vi "Move(X)feet.vi"(3 "Target":dbl, 5 "RobotDriveDevRef":T1={"DevStatus"={"status"=FALSE, "code"=0, "source"=""}, "Motors[]"=[], "Square Inputs"=FALSE, "Max Output"=1.0}, 6 "AccelerometerDevRef":T7={"DevStatus"={"status"=FALSE, "code"=0, "source"=""}, "Scaling"={"Gain (VoltsPerG)"=0.0, "Center Voltage"=0.0}, "Analog Channels"={"X-Axis"=enum."Invalid", "Y-Axis"=enum."Invalid", "Z-Axis"=enum."Invalid"}, "I2C Bus"=enum."Invalid", "SPI Bus"=enum."Invalid", "Accel Range"=0, "ADXL Axes"={"X-Axis"=FALSE, "Y-Axis"=FALSE, "Z-Axis"=FALSE}, "Handle"=0, "Device Address"=0, "Accel Type"=enum."Analog"} {"Device Address" format="%.0x"; "Accel Range" items=["+/- 2 g", "+/- 4 g", "+/- 8 g", "+/- 16 g"]}) -> (1 "RobotDriveDevRef":T1={"DevStatus"={"status"=FALSE, "code"=0, "source"=""}, "Motors[]"=[], "Square Inputs"=FALSE, "Max Output"=1.0}, 2 "AccelerometerDevRef":T7={"DevStatus"={"status"=FALSE, "code"=0, "source"=""}, "Scaling"={"Gain (VoltsPerG)"=0.0, "Center Voltage"=0.0}, "Analog Channels"={"X-Axis"=enum."Invalid", "Y-Axis"=enum."Invalid", "Z-Axis"=enum."Invalid"}, "I2C Bus"=enum."Invalid", "SPI Bus"=enum."Invalid", "Accel Range"=0, "ADXL Axes"={"X-Axis"=FALSE, "Y-Axis"=FALSE, "Z-Axis"=FALSE}, "Handle"=0, "Device Address"=0, "Accel Type"=enum."Analog"} {"Device Address" format="%.0x"; "Accel Range" items=["+/- 2 g", "+/- 4 g", "+/- 8 g", "+/- 16 g"]})   [LabVIEW 2017]
uses:
  <vilib>/Rock Robotics/WPI/Accelerometer/WPI_AccelerometerDevRef.ctl
  <vilib>/Rock Robotics/WPI/Accelerometer/WPI_AccelerometerScaling.ctl
  <vilib>/Rock Robotics/WPI/Accelerometer/WPI_AccelerometerAnalogChannels.ctl
  <vilib>/Rock Robotics/SystemInterfaces/AI/FPGA_AIChannel.ctl
  <vilib>/Rock Robotics/SystemInterfaces/i2clib/i2c_bus.ctl
  <vilib>/Rock Robotics/SystemInterfaces/spilib/spi_bus.ctl
  <vilib>/Rock Robotics/WPI/Accelerometer/ADXL345 Range.ctl
  <vilib>/Rock Robotics/WPI/Accelerometer/WPI_AccelerometerADXL345 Axes.ctl
  <vilib>/Rock Robotics/WPI/RobotDrive/WPI_RobotDriveDevRef.ctl
  <vilib>/Rock Robotics/WPI/MotorControl/WPI_MotorControlDeviceRef.ctl
  <vilib>/Rock Robotics/WPI/MotorControl/WPI_MotorControlType.ctl
  <vilib>/Rock Robotics/SystemInterfaces/DIO/FPGA_DIOPWMChannel.ctl
  <vilib>/Rock Robotics/WPI/PWM/WPI_PWMDeadband.ctl
  <vilib>/Rock Robotics/SystemInterfaces/DIO/FPGA_DIOChannel.ctl
  <vilib>/Rock Robotics/WPI/RobotDrive/WPI_RobotDriveArcadeDrive_Standard(NoSaturation).vi
  <vilib>/Rock Robotics/Network Tables/NT Write Number.vi
  <vilib>/Rock Robotics/Network Tables/NT Write Numeric Array.vi
panel:
  in  "Speed":dbl
  in  "Velocity":dbl
  in  "Distance":dbl
  in  "Start Time":dbl
  # "ADXL"
  # "Analog"
  # "ADXL"
  # "Analog"
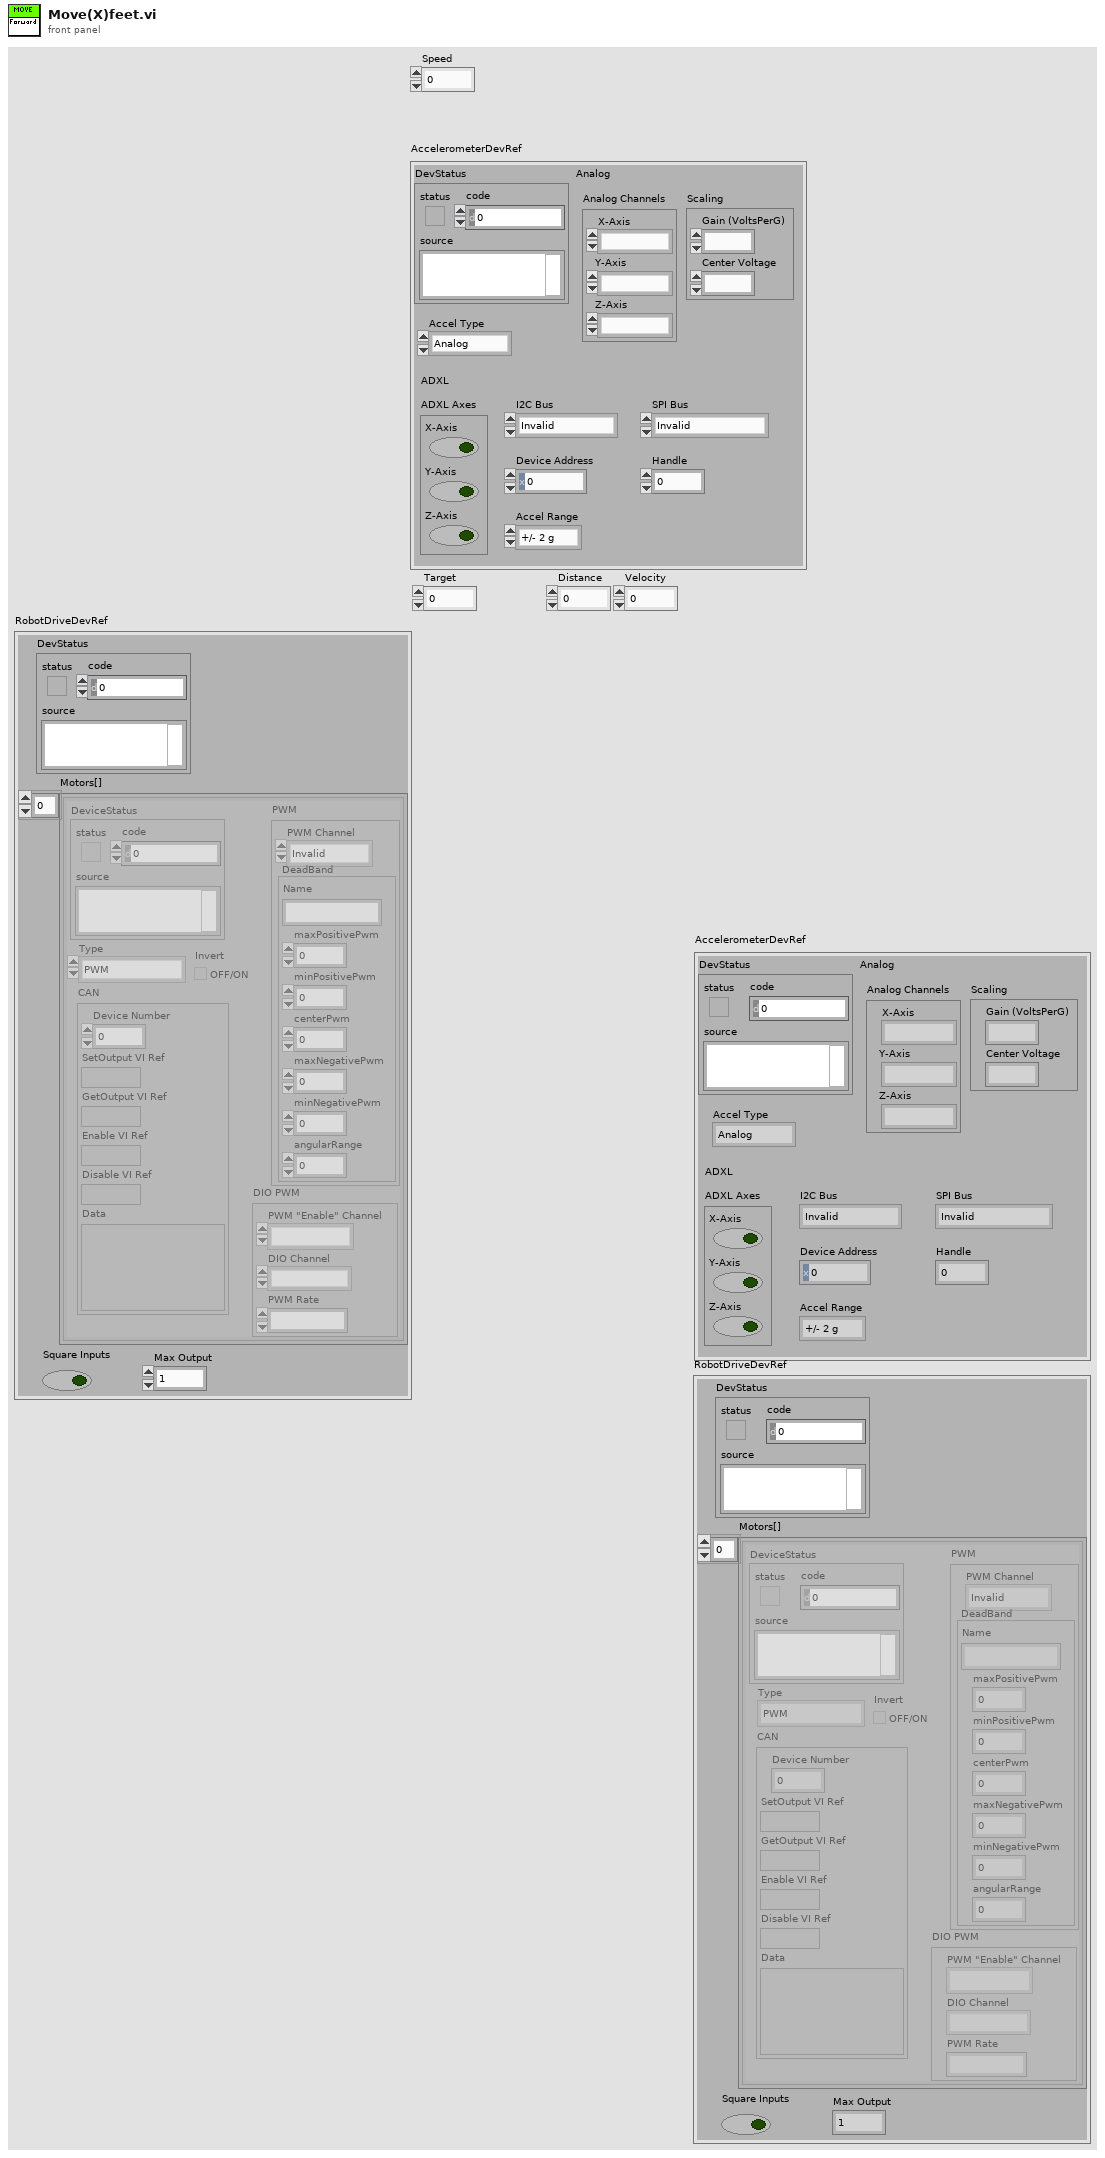
[diagram p1: front panel]
types:
  T1 = typedef "WPI_RobotDriveDevRef.ctl" = cluster{"DevStatus":errorcluster, "Motors[]":T2[], "Square Inputs":bool, "Max Output":dbl}
  T2 = typedef "WPI_MotorControlDeviceRef.ctl" = cluster{"DeviceStatus":errorcluster, "Type":T3, "PWM":cluster{"PWM Channel":T4, "DeadBand":T5}, "CAN":cluster{"Device Number":u8, "SetOutput VI Ref":variant, "GetOutput VI Ref":variant, "Enable VI Ref":variant, "Disable VI Ref":variant, "Data":variant}, "Invert":bool, "DIO PWM":cluster{"PWM \"Enable\" Channel":T4, "DIOChannel":T6, "PWM Rate":dbl}}
  T3 = typedef "WPI_MotorControlType.ctl" = enum16{"PWM", "CAN", "DIO PWM"}
  T4 = typedef "FPGA_DIOPWMChannel.ctl" = enum8{"PWM 0", "PWM 1", "PWM 2", "PWM 3", "PWM 4", "PWM 5", "PWM 6", "PWM 7", "PWM 8", "PWM 9", "PWM MXP 0", "PWM MXP 1", "PWM MXP 2", "PWM MXP 3", "PWM MXP 4", "PWM MXP 5", "PWM MXP 6", "PWM MXP 7", "PWM MXP 8", "PWM MXP 9", "Invalid"}
  T5 = typedef "WPI_PWMDeadband.ctl" = cluster{"Name":string, "maxPositivePwm":i32, "minPositivePwm":i32, "centerPwm":i32, "maxNegativePwm":i32, "minNegativePwm":i32, "angularRange":u16}
  T6 = typedef "FPGA_DIOChannel.ctl" = enum8{"DIO 0", "DIO 1", "DIO 2", "DIO 3", "DIO 4", "DIO 5", "DIO 6", "DIO 7", "DIO 8", "DIO 9", "DIO MXP 0", "DIO MXP 1", "DIO MXP 2", "DIO MXP 3", "DIO MXP 4", "DIO MXP 5", "DIO MXP 6", "DIO MXP 7", "DIO MXP 8", "DIO MXP 9", "DIO MXP 10", "DIO MXP 11", "DIO MXP 12", "DIO MXP 13", "DIO MXP 14", "DIO MXP 15", "SPI Port CS1", "SPI Port CS2", "SPI Port CS3", "SPI Port MISO", "SPI Port MOSI", "Invalid"}
  T7 = typedef "WPI_AccelerometerDevRef.ctl" = cluster{"DevStatus":errorcluster, "Scaling":T8, "Analog Channels":T9, "I2C Bus":T11, "SPI Bus":T12, "Accel Range":T13, "ADXL Axes":T14, "Handle":i32, "Device Address":u8, "Accel Type":enum16{"Analog", "ADXL345 I2C", "ADXL345 SPI", "Internal", "ADXL362 SPI"}}
  T8 = typedef "WPI_AccelerometerScaling.ctl" = cluster{"Gain (VoltsPerG)":dbl, "Center Voltage":dbl}
  T9 = typedef "WPI_AccelerometerAnalogChannels.ctl" = cluster{"X-Axis":T10, "Y-Axis":T10, "Z-Axis":T10}
  T10 = typedef "FPGA_AIChannel.ctl" = enum8{"AI 0", "AI 1", "AI 2", "AI 3", "AI MXP 0", "AI MXP 1", "AI MXP 2", "AI MXP 3", "Invalid"}
  T11 = typedef "i2c_bus.ctl" = enum16{"I2C On-Board", "I2C MXP", "Invalid"}
  T12 = typedef "spi_bus.ctl" = enum16{"SPI On-Board, CS0", "SPI On-Board, CS1", "SPI On-Board, CS2", "SPI On-Board, CS3", "SPI MXP", "Invalid"}
  T13 = typedef "ADXL345 Range.ctl" = u8
  T14 = typedef "WPI_AccelerometerADXL345 Axes.ctl" = cluster{"X-Axis":bool, "Y-Axis":bool, "Z-Axis":bool}
  T15 = cluster{"X-Axis":dbl, "Y-Axis":dbl, "Z-Axis":dbl}
  T16 = cluster{"Target":dbl, "Distance":dbl, dbl, dbl, dbl}
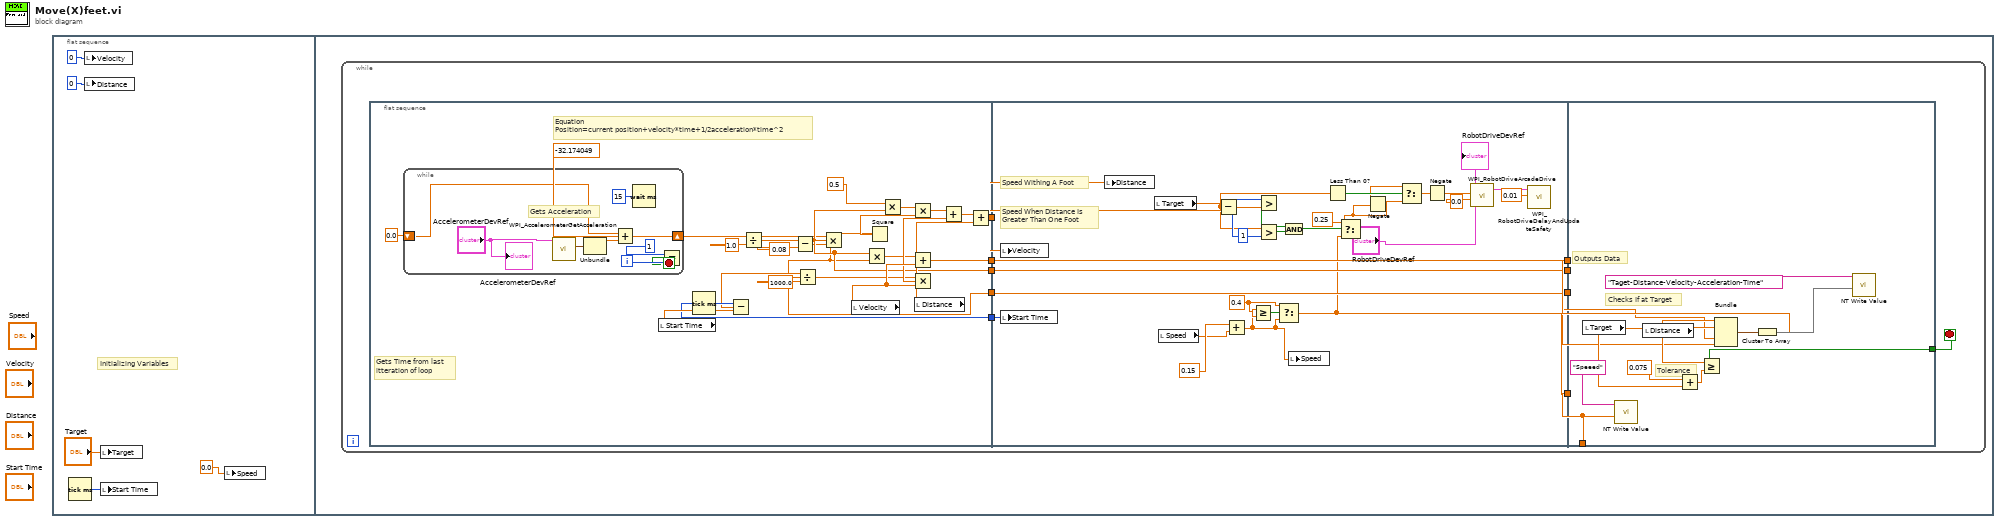
[diagram p0: block diagram]
diagram:
  n1 = flat-sequence {
    frame #0 {
      # "Initializing Variables"
      n2 = Tick Count (ms)() -> (millisecond timer value=w5:u32)
      n3 = local write "Velocity"(0) -> ()
      n4 = local write "Distance"(0) -> ()
      n5 = local write "Target"("Target") -> ()
      n6 = local write "Start Time"(w5) -> ()
      n7 = local write "Speed"(0.0) -> ()
    }
    frame #1 {
      n8 = while {
        stop <- w12 stop-if-true
        n9 = flat-sequence {
          tunnel: [w30] -> w15
          tunnel: [w29] -> w14
          tunnel: [w28] -> w13
          tunnel: [w27] -> w10
          tunnel: [w22] -> w8
          tunnel: w15 -> [w63]
          tunnel: w14 -> [w75]
          tunnel: w13 -> [w73]
          tunnel: [w63] -> w11
          tunnel: w10 -> [w62]
          tunnel: [w62] -> w9
          tunnel: w8 -> [w58]
          tunnel: [w58] -> w7
          tunnel: [w54] -> w6
          tunnel: [w87] -> w12
          tunnel: w11 -> [w80]
          tunnel: w9 -> [w79]
          tunnel: w7 -> [w78]
          tunnel: w6 -> [w76]
          tunnel: [w76] -> _
          frame #0 {
            # "Gets Time from last \nitteration of loop"
            # "Equation\nPosition=current position+velocity*time+1/2acceleration*time^2"
            n10 = while {
              shift-right: [w44] -> w19
              shift-left: 0.0 -> [w43]
              i -> [w47]
              stop <- w45 stop-if-true
              # "Gets Acceleration"
              n11 = call <vilib>:"WPI_AccelerometerGetAcceleration.vi"("AccelerometerDevRef"="AccelerometerDevRef") -> ("Accelerations"=w48:T15)  [unwired: 8 in, 2 out]
              n12 = Unbundle(w48) -> ("Y-Axis"=w42:dbl)  [unwired: 2 out]
              n13 = Add(x=w43, y=w42) -> (x+y=w44:dbl)
              n14 = Wait (ms)(milliseconds to wait=u32 15) -> ()  [unwired: 1 out]
              n15 = Equal?(x=1, y=w47) -> (x = y?=w45:bool)
              "AccelerometerDevRef" <- "AccelerometerDevRef"
            }
            n16 = local read "Start Time"() -> (w39:dbl)
            n17 = Tick Count (ms)() -> (millisecond timer value=w29:u32)
            n18 = Subtract(x=w29, y=w39) -> (x-y=w25:dbl)
            n19 = Divide(x=w19, y=1.0) -> (x/y=w17:dbl)
            n20 = Subtract(x=w17, y=0.08) -> (x-y=w20:dbl)
            n21 = Divide(x=w25, y=1000.0) -> (x/y=w22:dbl)
            n22 = Multiply(x=-32.174049, y=w20) -> (x*y=w27:dbl)
            n23 = local read "Velocity"() -> (w34:dbl)
            n24 = Multiply(x=w27, y=w22) -> (x*y=w26:dbl)
            n25 = Square(x=w22) -> (x^2=w36:dbl)
            n26 = Multiply(x=0.5, y=w27) -> (x*y=w38:dbl)
            n27 = Multiply(x=w38, y=w36) -> (x*y=w32:dbl)
            n28 = Add(x=w26, y=w34) -> (x+y=w30:dbl)
            n29 = Multiply(x=w22, y=w34) -> (x*y=w33:dbl)
            n30 = local read "Distance"() -> (w35:dbl)
            n31 = Add(x=w32, y=w33) -> (x+y=w31:dbl)
            n32 = Add(x=w31, y=w35) -> (x+y=w28:dbl)
          }
          frame #1 {
            w56 = 0.4 ("t")
            w72 = 1
            # "Speed When Distance Is \nGreater Than One Foot"
            # "Speed Withing A Foot"
            n33 = local write "Velocity"(w63) -> ()
            n34 = local write "Start Time"(w75) -> ()
            n35 = local write "Distance"(w73) -> ()
            n36 = local read "Target"() -> (w74:dbl)
            n37 = local read "Speed"() -> (w53:dbl)
            n38 = Subtract(x=w74, y=w73) -> (x-y=w67:dbl)
            n39 = Add(x=0.15, y=w53) -> (x+y=w50:dbl)
            n40 = Greater Or Equal?(x=w50, y=w56) -> (x >= y?=w57:bool)
            n41 = Greater?(x=w72, y=w67) -> (0:w71:bool)
            n42 = Greater?(x=w67, y=w72) -> (0:w70:bool)
            n43 = Select(t=w56, s=w57, f=w50) -> (s? t:f=w54:dbl)
            n44 = And(x=w71, y=w70) -> (x .and. y?=w69:bool)
            n45 = local write "Speed"(w50) -> ()
            n46 = Less Than 0?(x=w67) -> (x < 0?=w66:bool)
            n47 = Select(t=0.25, s=w69, f=w54) -> (s? t:f=w65:dbl)
            n48 = Negate(x=w65) -> (-x=w64:dbl)
            n49 = Select(t=w64, s=w66, f=w65) -> (s? t:f=w60:dbl)
            n50 = Negate(x=w60) -> (-x=w61:dbl)
            n51 = call-poly <vilib>:"WPI_RobotDriveArcadeDrive.vi"("Y axis value"=0.0, "X axis value"=w61, "RobotDriveDevRef"="RobotDriveDevRef") -> ("RobotDriveDevRef"=w52:T1)  [unwired: 6 in, 2 out]
            n52 = call <vilib>:"WPI_RobotDriveDelayAndUpdateSafety.vi"("Delay (s)"=0.01, "RobotDriveDevRef"=w52) -> ()  [unwired: 8 in, 2 out]
            "RobotDriveDevRef" <- "RobotDriveDevRef"
          }
          frame #2 {
            # "Tolerance"
            # "Checks If at Target"
            # "Outputs Data"
            n53 = local read "Target"() -> (w85:dbl)
            n54 = call-poly <vilib>:"NT Write Value.vi"("Numeric"=w76, "Name"="Speeed") -> ()  [unwired: 9 in, 1 out]
            n55 = local read "Distance"() -> (w84:dbl)
            n56 = Add(x=0.075, y=w85) -> (x+y=w88:dbl)
            n57 = Greater Or Equal?(x=w84, y=w88) -> (x >= y?=w87:bool)
            n58 = Bundle("Target"=w85, "Distance"=w84, w80, w79, w78) -> (w83:T16)  [unwired: 1 in]
            n59 = Cluster To Array(cluster=w83) -> (array=w82:dbl[])
            n60 = call-poly <vilib>:"NT Write Value.vi"("Numeric Array"=w82, "Name"="Taget-Distance-Velocity-Acceleration-Time") -> ()  [unwired: 9 in, 1 out]
          }
        }
      }
    }
  }
